vi "Untitled 5 (SubVI).vi"(11 "Array in":dbl[](array[numeric])) -> (3 "Array":dbl[](array[numeric]))   [LabVIEW 2017]
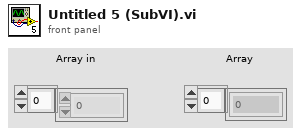
[diagram p1: front panel]
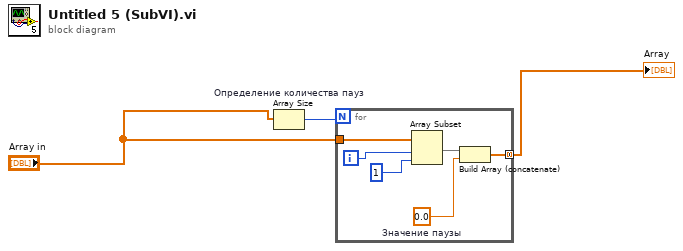
[diagram p0: block diagram]
diagram:
  n1 = Array Size "Определение количества пауз"(array="Array in") -> (size(s)=w1:i32)
  n2 = for {
    N: w1 -> [_]
    tunnel: "Array in" -> [w6]
    tunnel: [w5] -> w3 mode=concatenating
    i -> [w4]
    w7 = 0.0  # Значение паузы
    n3 = Array Subset(array=w6, index=w4, length=1) -> (w8:dbl[])
    n4 = Build Array (concatenate)(w8, w7) -> (w5:dbl[])
  }
  "Array" <- w3
